vi "OE1022D Example All Data.vi"() -> ()   [LabVIEW 2022 SP3]
uses:
  <vilib>/Utility/file.llb/Write Delimited Spreadsheet (DBL).vi
panel:
  out "Waveform Chart":dbl[](graph)
  in  "Path 2":path
  in  "Stop":bool
  out "θh1 (°) 2":sgl caption="θh1 (deg)" format="%.2f"
  out "Rh1 2":sgl caption="Rh1 (Vrms)" format="%.3p"
  out "Yh1 2":sgl caption="Yh1 (Vrms)" format="%.3p"
  out "Xh1 2":sgl caption="Xh1 (Vrms)" format="%.3p"
  out "Xh2 2":sgl caption="Xh2 (Vrms)" format="%.3p"
  out "Yh2 2":sgl caption="Yh2 (Vrms)" format="%.3p"
  out "Rh2 2":sgl caption="Rh2 (Vrms)" format="%.3p"
  out "噪声 2":sgl caption="Noise(Vrms)" format="%.3p"
  out "频率 (Hz) 2":sgl caption="Freq (Hz)" format="%#.3f"
  out "θ (°) 2":sgl caption="θ (deg)" format="%.2f"
  out "R 2":sgl caption="R (Vrms)" format="%.3p"
  out "Y 2":sgl caption="Y (Vrms)" format="%.3p"
  out "θh2 (°) 2":sgl caption="θh2 (deg)" format="%.2f"
  out "X 2":sgl caption="X (Vrms)" format="%.3p"
  out "Yh1":sgl caption="Yh1 (Vrms)" format="%.3p"
  out "Xh1":sgl caption="Xh1 (Vrms)" format="%.3p"
  out "θh2 (°)":sgl caption="θh2 (deg)" format="%.2f"
  out "Yh2":sgl caption="Yh2 (Vrms)" format="%.3p"
  out "Xh2":sgl caption="Xh2 (Vrms)" format="%.3p"
  out "Rh2":sgl caption="Rh2 (Vrms)" format="%.3p"
  out "θh1 (°)":sgl caption="θh1 (deg)" format="%.2f"
  out "Rh1":sgl caption="Rh1 (Vrms)" format="%.3p"
  out "噪声":sgl caption="Noise(Vrms)" format="%.3p"
  out "频率 (Hz)":sgl caption="Freq (Hz)" format="%#.3f"
  out "θ (°)":sgl caption="θ (deg)" format="%.2f"
  out "Y":sgl caption="Y (Vrms)" format="%.3p"
  out "X":sgl caption="X (Vrms)" format="%.3p"
  out "R":sgl caption="R (Vrms)" format="%.3p"
  out "AUX-ADC2 (V)":sgl format="%.3f"
  out "AUX-ADC1 (V)":sgl format="%.3f"
  out "AUX-ADC3 (V)":sgl format="%.3f"
  out "AUX-ADC4 (V)":sgl format="%.3f"
  out "错误输出":errorcluster
  out "序列号":string
  in  "OE1022D":refnum<visa-resource-name>
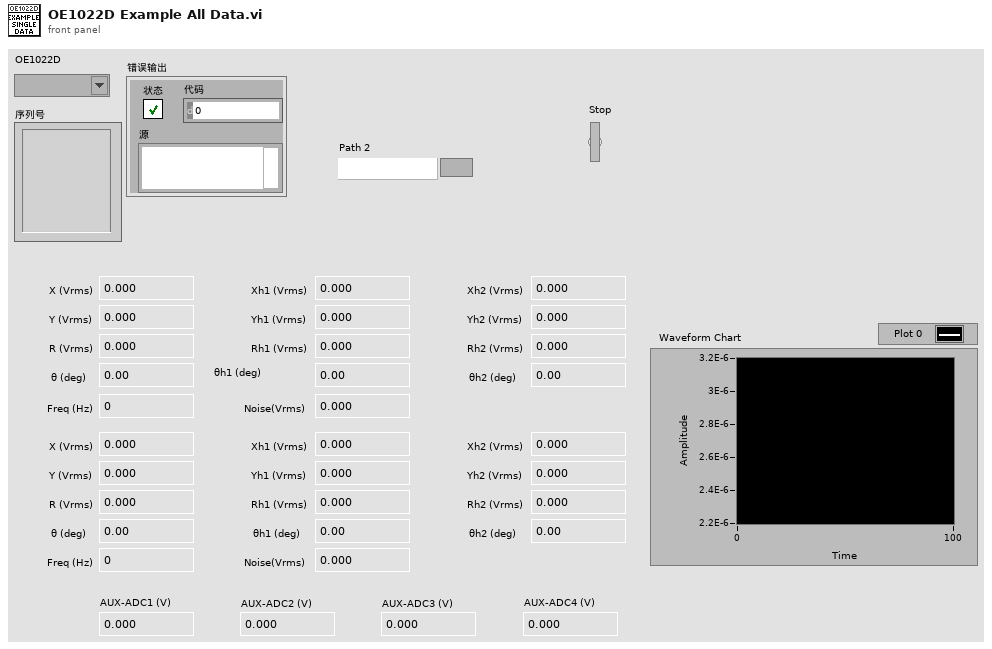
[diagram p1: front panel]
types:
  T1 = cluster{"AD1":dbl[], "AD2":dbl[], "AD3":dbl[], "AD4":dbl[]}
  T2 = cluster{"XB":dbl[], "YB":dbl[], "FrequencyB":dbl[], "NoiseB":dbl[], "Xh1B":dbl[], "Yh1B":dbl[], "Xh2B":dbl[], "Yh2B":dbl[], "Xh2B":dbl[]}
  T3 = cluster{"XA":dbl[], "YA":dbl[], "FrequencyA":dbl[], "NoiseA":dbl[], "Xh1A":dbl[], "Yh1A":dbl[], "Xh2A":dbl[], "Yh2A":dbl[]}
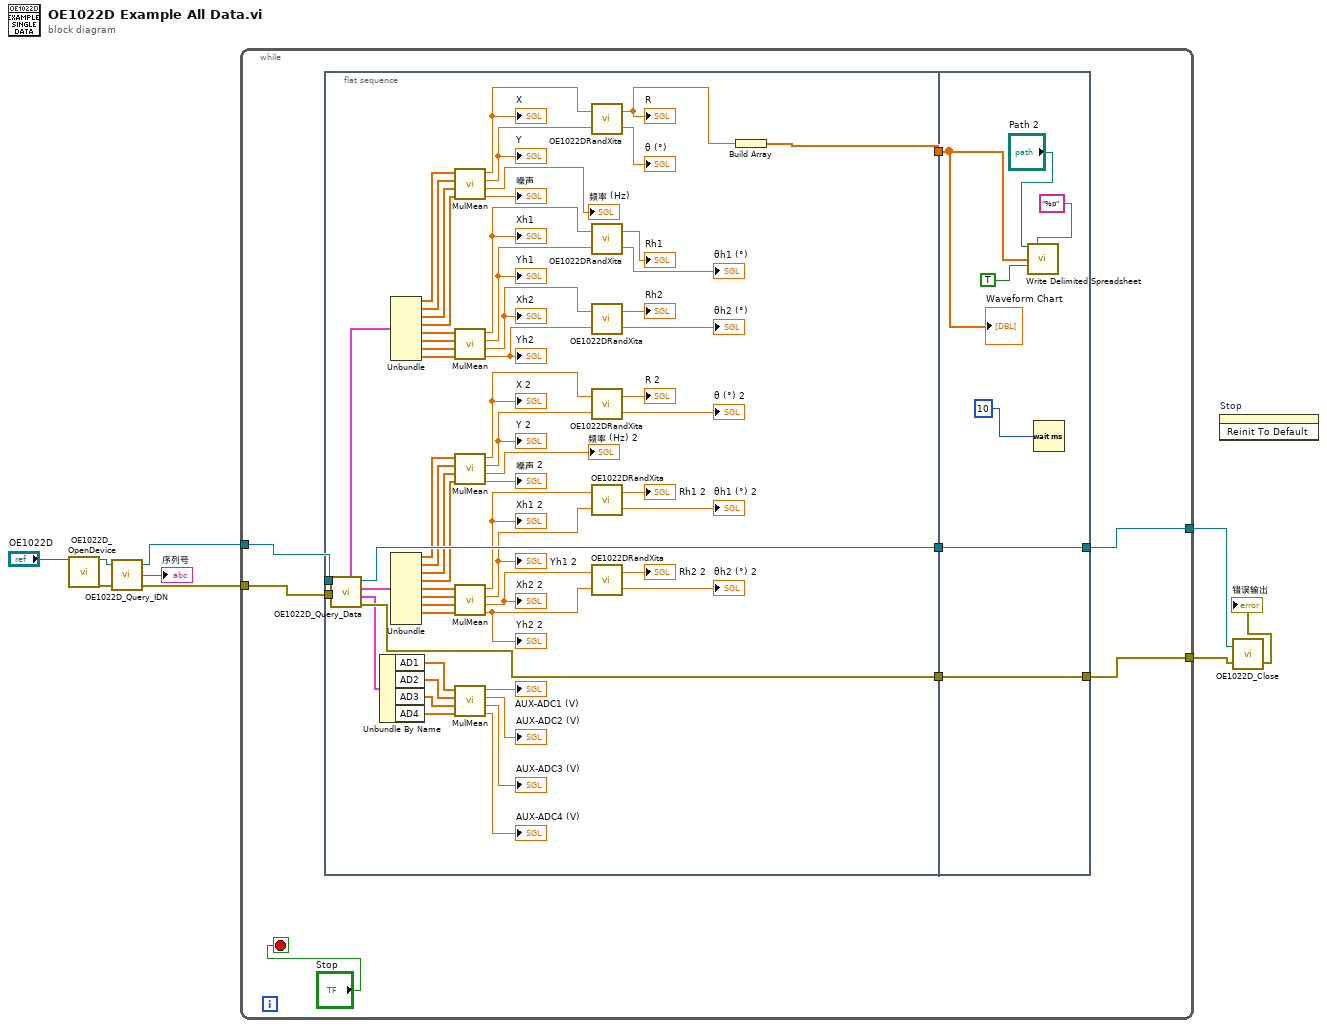
[diagram p0: block diagram]
diagram:
  n1 = call "OE1022D_OpenDevice.vi"("VISA resource name"="OE1022D") -> ("VISA资源名称输出"=w6:refnum<visa-resource-name>, "错误输出"=w7:errorcluster)  [unwired: 17 in]
  n2 = call "OE1022D_Query_IDN.vi"("错误输入（无错误）"=w7, "VISA resource name"=w6) -> ("错误输出"=w5:errorcluster, "序列号"=→"序列号":string, "VISA resource name out"=w4:refnum<visa-resource-name>)  [unwired: 1 in]
  n3 = while {
    tunnel: w5 -> [w17]
    tunnel: w4 -> [w16]
    tunnel: [w15] -> w3
    tunnel: [w14] -> w2
    stop <- "Stop" stop-if-true
    n4 = flat-sequence {
      tunnel: w17 -> [w77]
      tunnel: w16 -> [w76]
      tunnel: [w75] -> w12
      tunnel: [w74] -> w11
      tunnel: [w73] -> w10
      tunnel: [w83] -> w14
      tunnel: [w84] -> w15
      tunnel: w12 -> [w84]
      tunnel: w11 -> [w83]
      tunnel: w10 -> [w81]
      frame #0 {
        n5 = call "OE1022D_Query_Data.vi"("错误输入（无错误）"=w77, "VISA resource name"=w76) -> ("error out"=w75:errorcluster, "输出簇ADC"=w20:T1, "输出簇B"=w19:T2, "VISA resource name out"=w74:refnum<visa-resource-name>, "输出簇A"=w21:T3)  [unwired: 3 in]
        n6 = Unbundle By Name(w20) -> ("AD1"=w69:dbl[], "AD2"=w70:dbl[], "AD3"=w71:dbl[], "AD4"=w72:dbl[])
        n7 = Unbundle(w21) -> ("XA"=w26:dbl[], "YA"=w27:dbl[], "FrequencyA"=w28:dbl[], "NoiseA"=w29:dbl[], "Xh1A"=w35:dbl[], "Yh1A"=w36:dbl[], "Xh2A"=w37:dbl[], "Yh2A"=w38:dbl[])
        n8 = Unbundle(w19) -> ("XB"=w54:dbl[], "YB"=w53:dbl[], "FrequencyB"=w52:dbl[], "NoiseB"=w51:dbl[], "Xh1B"=w50:dbl[], "Yh1B"=w49:dbl[], "Xh2B"=w48:dbl[], "Yh2B"=w47:dbl[])  [unwired: 1 out]
        n9 = call "MulMean.vi"("IN 4"=w29, "IN 3"=w28, "IN 2"=w27, "IN 1"=w26) -> ("mean 4"=→"噪声":dbl, "mean 3"=→"频率 (Hz)":dbl, "mean 2"=w32:dbl, "mean 1"=w31:dbl)  [unwired: 4 in]
        "X" <- w31
        "Y" <- w32
        n10 = call "MulMean.vi"("IN 4"=w38, "IN 3"=w37, "IN 2"=w36, "IN 1"=w35) -> ("mean 4"=w44:dbl, "mean 3"=w43:dbl, "mean 2"=w40:dbl, "mean 1"=w39:dbl)  [unwired: 4 in]
        "Xh2" <- w43
        "Yh2" <- w44
        "Xh1" <- w39
        "Yh1" <- w40
        n11 = call "MulMean.vi"("IN 4"=w51, "IN 3"=w52, "IN 2"=w53, "IN 1"=w54) -> ("mean 4"=→"噪声 2":dbl, "mean 3"=→"频率 (Hz) 2":dbl, "mean 2"=w60:dbl, "mean 1"=w59:dbl)  [unwired: 4 in]
        "X 2" <- w59
        "Y 2" <- w60
        n12 = call "MulMean.vi"("IN 4"=w47, "IN 3"=w48, "IN 2"=w49, "IN 1"=w50) -> ("mean 4"=w66:dbl, "mean 3"=w65:dbl, "mean 2"=w62:dbl, "mean 1"=w61:dbl)  [unwired: 4 in]
        "Yh2 2" <- w66
        "Xh2 2" <- w65
        "Xh1 2" <- w61
        "Yh1 2" <- w62
        n13 = call "MulMean.vi"("IN 4"=w72, "IN 3"=w71, "IN 2"=w70, "IN 1"=w69) -> ("mean 4"=→"AUX-ADC4 (V)":dbl, "mean 3"=→"AUX-ADC3 (V)":dbl, "mean 2"=→"AUX-ADC2 (V)":dbl, "mean 1"=→"AUX-ADC1 (V)":dbl)  [unwired: 4 in]
        n14 = call "OE1022DRandXita.vi"("Y"=w32, "X"=w31) -> ("θ (°)"=→"θ (°)":dbl, "R"=w18:dbl)
        "R" <- w18
        n15 = call "OE1022DRandXita.vi"("Y"=w40, "X"=w39) -> ("θ (°)"=→"θh1 (°)":dbl, "R"=→"Rh1":dbl)
        n16 = call "OE1022DRandXita.vi"("Y"=w44, "X"=w43) -> ("θ (°)"=→"θh2 (°)":dbl, "R"=→"Rh2":dbl)
        n17 = call "OE1022DRandXita.vi"("Y"=w60, "X"=w59) -> ("θ (°)"=→"θ (°) 2":dbl, "R"=→"R 2":dbl)
        n18 = call "OE1022DRandXita.vi"("Y"=w62, "X"=w61) -> ("θ (°)"=→"θh1 (°) 2":dbl, "R"=→"Rh1 2":dbl)
        n19 = call "OE1022DRandXita.vi"("Y"=w66, "X"=w65) -> ("θ (°)"=→"θh2 (°) 2":dbl, "R"=→"Rh2 2":dbl)
        n20 = Build Array(w18) -> (w73:dbl[])
      }
      frame #1 {
        n21 = call-poly <vilib>:"Write Delimited Spreadsheet.vi"("file path (dialog if empty)"="Path 2", "format (%.3f)"="%p", "1D data"=w81, "append to file? (new file:F)"=TRUE) -> ()  [unwired: 10 in, 2 out]
        n22 = Wait (ms)(milliseconds to wait=10) -> ()  [unwired: 1 out]
        "Waveform Chart" <- w81
      }
    }
  }
  n23 = invoke on="Stop" class="Bool (strict)" method="Reinit To Default"() -> ()  [unwired: 3 in, 3 out]
  n24 = call "OE1022D_Close.vi"("错误输入（无错误）"=w3, "VISA resource name"=w2) -> ("错误输出"=→"错误输出":errorcluster)  [unwired: 1 in]
